vi "Add_file_count.vi"() -> ()   [LabVIEW 2019]
uses:
  Global Variables/Data_Display_global.vi
panel:
  out "Path":path
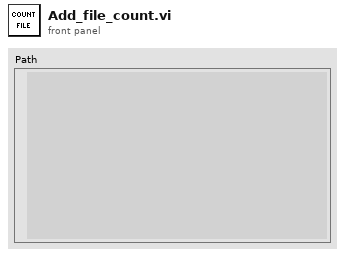
[diagram p1: front panel]
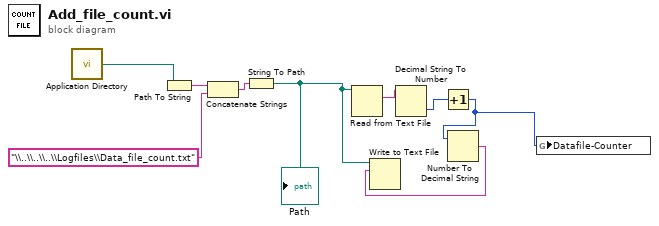
[diagram p0: block diagram]
diagram:
  n1 = call <vilib>:"Application Directory.vi"() -> ("Application Directory"=w5:path)
  n2 = Path To String(path=w5) -> (string=w4:string)
  n3 = Concatenate Strings(w4, "\\..\\..\\..\\Logfiles\\Data_file_count.txt") -> (w3:string)
  n4 = String To Path(string=w3) -> (path=w2:path)
  "Path" <- w2
  n5 = Read from Text File(file (use dialog)=w2) -> (text=w9:string)  [unwired: 3 in, 3 out]
  n6 = Decimal String To Number(string=w9) -> (number=w8:i32)  [unwired: 2 in, 1 out]
  n7 = Increment(x=w8) -> (x+1=w6:i32)
  n8 = Number To Decimal String(number=w6) -> (decimal integer string=w7:string)  [unwired: 1 in]
  n9 = Write to Text File(file (use dialog)=w2, text=w7) -> ()  [unwired: 2 in, 3 out]
  n10 = global write "Data_Display_global.vi" "Datafile-Counter"(w6) -> ()
